vi "Handle TCP Message.vi"(7 "TCPMessageAPI":refnum<class "TCPMessageAPI.lvclass">, 8 "error in (no error)":errorcluster, 10 "TcpPayload":T1, 11 "TCPMessageHandler in":refnum<class "TCPMessageHandler.lvclass">) -> (0 "error out":errorcluster, 3 "TCPMessageHandler out":refnum<class "TCPMessageHandler.lvclass">)   [LabVIEW 2020, in "Vecto.lvlib" / "TCPMessageHandler.lvclass"]
uses:
  TCPMessageHandler.lvclass
  TCPMessageService/TCPMessageAPI.lvclass
  lv-volatus/messages/TcpPayload/Data.ctl
  lv-volatus/messages/TcpPayload/TcpPayload.lvlib
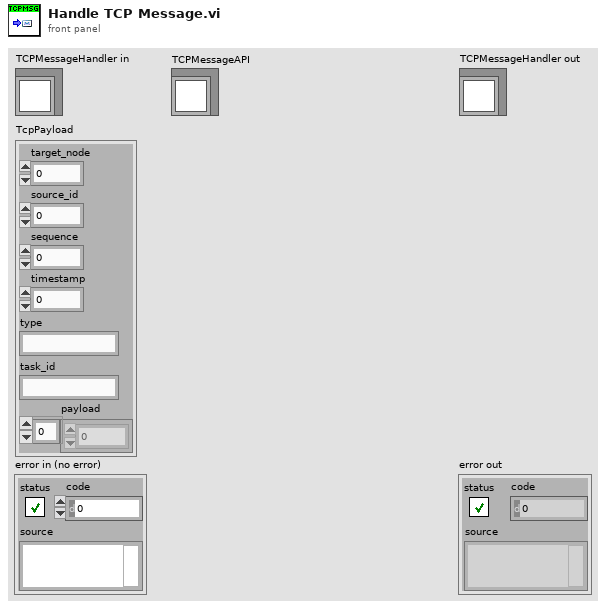
[diagram p1: front panel]
types:
  T1 = typedef "TcpPayload.lvlib/Data.ctl" = cluster{"target_node":u32, "source_id":u32, "sequence":u32, "timestamp":i64, "type":string, "task_id":string, "payload":u8[]}
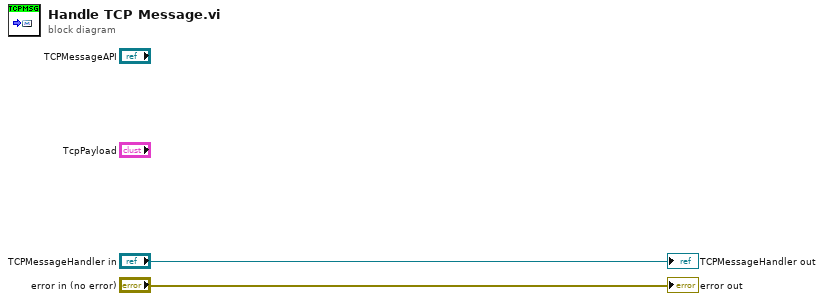
[diagram p0: block diagram]
diagram:
  "error out" <- "error in (no error)"
  "TCPMessageHandler out" <- "TCPMessageHandler in"
